vi "_038.vi"() -> ()   [LabVIEW 2024]
panel:
  out "s? t:f 3":string
  out "s? t:f 2":string
  in  "Using Loops":i32
  out "s? t:f":string
  in  "Without using Loop":dbl
  # "Palindrome"
  # "( Using & Without using Loops )"
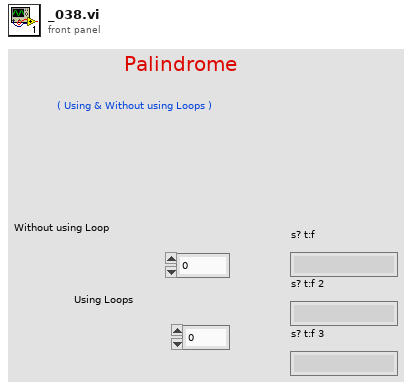
[diagram p1: front panel]
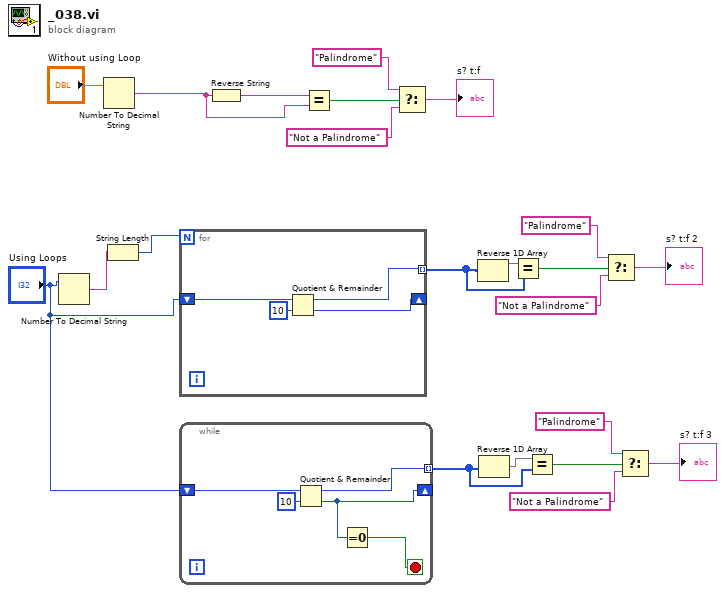
[diagram p0: block diagram]
diagram:
  n1 = Number To Decimal String(number="Using Loops") -> (decimal integer string=w15:string)  [unwired: 1 in]
  n2 = Number To Decimal String(number="Without using Loop") -> (decimal integer string=w20:string)  [unwired: 1 in]
  n3 = String Length(string=w15) -> (length=w14:i32)
  n4 = for {
    N: w14 -> [_]
    shift-right: [w23] -> _
    shift-left: "Using Loops" -> [w26]
    tunnel: [w25] -> w3 mode=indexing
    n5 = Quotient & Remainder(x=w26, y=10) -> (x-y*floor(x/y)=w25:i32, floor(x/y)=w23:i32)
  }
  n6 = while {
    shift-right: [w28] -> _
    shift-left: "Using Loops" -> [w31]
    tunnel: [w30] -> w1 mode=indexing
    stop <- w27 stop-if-true
    n7 = Quotient & Remainder(x=w31, y=10) -> (x-y*floor(x/y)=w30:i32, floor(x/y)=w28:i32)
    n8 = Equal To 0?(x=w28) -> (x = 0?=w27:bool)
  }
  n9 = Reverse String(1:w20) -> (0:w21:string)
  n10 = Equal?(x=w21, y=w20) -> (x = y?=w19:bool)
  n11 = Select(t="Palindrome", s=w19, f="Not a Palindrome") -> (s? t:f=→"s? t:f":string)
  n12 = Reverse 1D Array(array=w3) -> (reversed array=w4:i32[])
  n13 = Reverse 1D Array(array=w1) -> (reversed array=w2:i32[])
  n14 = Equal?(x=w4, y=w3) -> (x = y?=w9:bool)
  n15 = Equal?(x=w2, y=w1) -> (x = y?=w8:bool)
  n16 = Select(t="Palindrome", s=w9, f="Not a Palindrome") -> (s? t:f=→"s? t:f 2":string)
  n17 = Select(t="Palindrome", s=w8, f="Not a Palindrome") -> (s? t:f=→"s? t:f 3":string)
